vi "Convert State For Save.vi"(2 "Container State":T1, 3 "Display State":T2) -> (1 "Display State To Save":variant)   [LabVIEW 2020, in "3D Contour.xctl"]
uses:
  <vilib>/Math Plots/3D Math Plots/3D Contour/3D Contour XCtrl/3D Contour.xctl
  <vilib>/Math Plots/3D Math Plots/3D Contour/3D Contour XCtrl/State.ctl
  <vilib>/Math Plots/3D Math Plots/3D Contour/3D Contour/3D Contour.lvclass
  e:/builds/penguin/labview/branches/2020/dev/dist/vi.lib/Math Plots/3D Math Plots/3D Plot/3D Plot/3D Plot.lvclass
  <vilib>/Math Plots/3D Math Plots/3D Plot/Action String/3DMathPlot Ctrl Act Queue.ctl
  <vilib>/Math Plots/3D Math Plots/3D Plot/Action String/3DMathPlot Ctrl Act Cluster.ctl
  <vilib>/Math Plots/3D Math Plots/3D Plot/Action String/3DMathPlot State Class.ctl
  <vilib>/_xctls/Container State.ctl
  <vilib>/Math Plots/3D Math Plots/3D Plot/3D Plot/3D Plot.lvclass
  <vilib>/_xctls/XControlSupport.lvlib
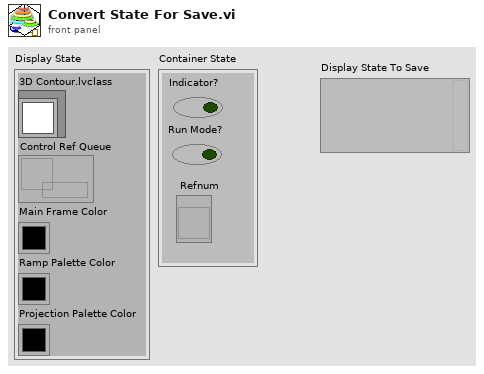
[diagram p1: front panel]
types:
  T1 = typedef "XControlSupport.lvlib/Container State.ctl" = cluster{"Indicator?":bool, "Run Mode?":bool, " Refnum":refnum<vi>}
  T2 = typedef "3D Contour.xctl/State.ctl" = cluster{"3D Contour.lvclass":refnum<class "3D Contour.lvclass">, "Control Ref Queue":T3, "Main Frame Color":u32, "Ramp Palette Color":u32, "Projection Palette Color":u32}
  T3 = typedef "3DMathPlot Ctrl Act Queue.ctl" = refnum<queue>
  T4 = enum32{"Towards X-Y Plane", "Towards X-Z Plane", "Towards Y-Z Plane", "User Defined"}
  T5 = typedef "3DMathPlot Ctrl Act Cluster.ctl" = cluster{"3D Picture Control":refnum<vi>, "Render Window Refnum":refnum<vi>, "XY Graph":refnum<vi>, "Intensity Graph":refnum<vi>, "Color Legend Palette":refnum<vi>, "Projection Palette":refnum<vi>, "XControl  Ref":refnum<vi>, "Facade Ref":refnum<vi>, "Export Image Ref":refnum<vi>, "Clear Data Flag":bool, "Display State Change Class":T6}
  T6 = typedef "3DMathPlot State Class.ctl" = enum16{"Update All Objects (Undo)", "Update Light Object Only", "Update Axis Object Only", "Update Plot Object Only", "Update Cursor Object Only", "Update Axis Plot Cursor Objects", "No Update"}
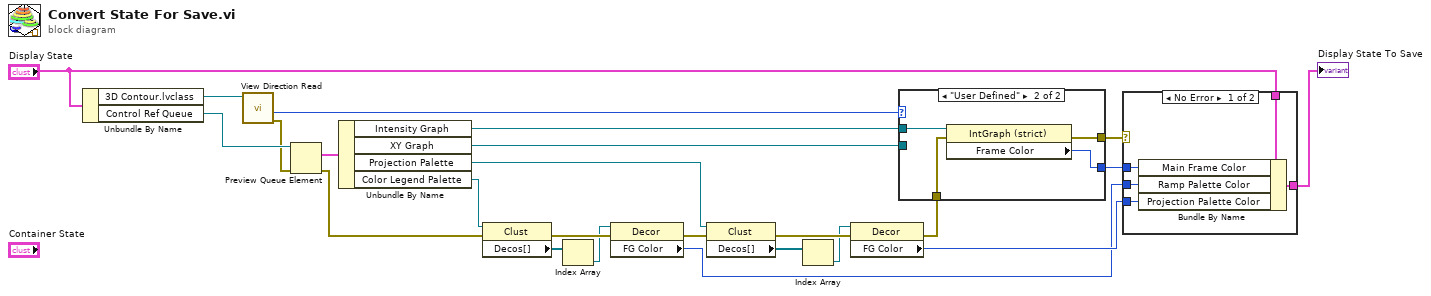
[diagram p0: block diagram]
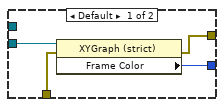
[diagram p3: hidden frame]
diagram:
  n1 = Unbundle By Name("Display State") -> ("3D Contour.lvclass"=w7:refnum<class "3D Contour.lvclass">, "Control Ref Queue"=w24:T3)
  n2 = call <vilib>:"View Direction Read.vi"("3D Plot.lvclass in"=w7) -> ("error out"=w4:errorcluster, "Value"=w6:T4)  [unwired: 8 in, 1 out]
  n3 = Preview Queue Element(queue=w24, error in (no error)=w4) -> (element=w23:T5, error out=w8:errorcluster)  [unwired: 3 out]
  n4 = Unbundle By Name(w23) -> ("Intensity Graph"=w5:refnum<vi>, "XY Graph"=w12:refnum<vi>, "Projection Palette"=w15:refnum<vi>, "Color Legend Palette"=w10:refnum<vi>)
  n5 = property class="Clust"(reference=w10, error in=w8) -> (error out=w20:errorcluster, "Decos[]"=w16:refnum<vi>[])  [unwired: 1 out]
  n6 = Index Array(array=w16) -> (element=w17:refnum<vi>)  [unwired: 1 in]
  n7 = property class="Decor"(reference=w17, error in=w20) -> (error out=w21:errorcluster, "FG Color"=w13:u32)  [unwired: 1 out]
  n8 = property class="Clust"(reference=w15, error in=w21) -> (error out=w22:errorcluster, "Decos[]"=w19:refnum<vi>[])  [unwired: 1 out]
  n9 = Index Array(array=w19) -> (element=w18:refnum<vi>)  [unwired: 1 in]
  n10 = property class="Decor"(reference=w18, error in=w22) -> (error out=w9:errorcluster, "FG Color"=w14:u32)  [unwired: 1 out]
  n11 = case shown="\"User Defined\"" w6 {
    tunnel: w12 -> [w28 _]
    tunnel: [w27 w30] -> w11
    tunnel: w9 -> [w26 w31]
    tunnel: w5 -> [_ w32]
    tunnel: [w25 w29] -> w1
    frame Default {
      n12 = property class="XYGraph (strict)"(reference=w28, error in=w26) -> (error out=w25:errorcluster, "Frame Color"=w27:u32)  [unwired: 1 out]
    }
    frame "User Defined" {
      n13 = property class="IntGraph (strict)"(reference=w32, error in=w31) -> (error out=w29:errorcluster, "Frame Color"=w30:u32)  [unwired: 1 out]
    }
  }
  n14 = case shown="No Error" w1 {
    tunnel: w14 -> [w37 _]
    tunnel: w13 -> [w36 _]
    tunnel: w11 -> [w35 _]
    tunnel: "Display State" -> [w34 w38]
    tunnel: [w33 w38] -> w2
    frame No Error {
      n15 = Bundle By Name(cluster=w34, "Main Frame Color"=w35, "Ramp Palette Color"=w36, "Projection Palette Color"=w37) -> (w33:T2)
    }
    frame Error {
    }
  }
  "Display State To Save" <- w2
